vi "MakeDoor.vi"(7 "DoorID":T1, 8 "error in (no error)":errorcluster, 9 "Room 2":refnum<class "Room.lvclass">, 10 "Room 1":refnum<class "Room.lvclass">, 11 "MazeGame":refnum<class "MazeGame.lvclass">) -> (0 "error out":errorcluster, 2 "Door":refnum<class "Door.lvclass">, 3 "MazeGame":refnum<class "MazeGame.lvclass">)   [LabVIEW 2020, in "FactoryMethod.lvlib" / "ParameterizedFactoryMethod.lvlib" / "MazeGame.lvclass"]
uses:
  MazeGame.lvclass
  GoFcommonClasses/ConcreteMazeSite/Room/Room.lvclass
  GoFcommonClasses/ConcreteMazeSite/Door/Door.lvclass
  TypeDef/DoorID.ctl
  GoFcommonClasses/ConcreteMazeSite/DoorNeedingSpell/DoorNeedingSpell.lvclass
  E:/Francesco/GitHub/Design-Patterns-GoF_-_NI-LV/Creational/GoFcommonClasses/ConcreteMazeSite/Door/Door.lvclass
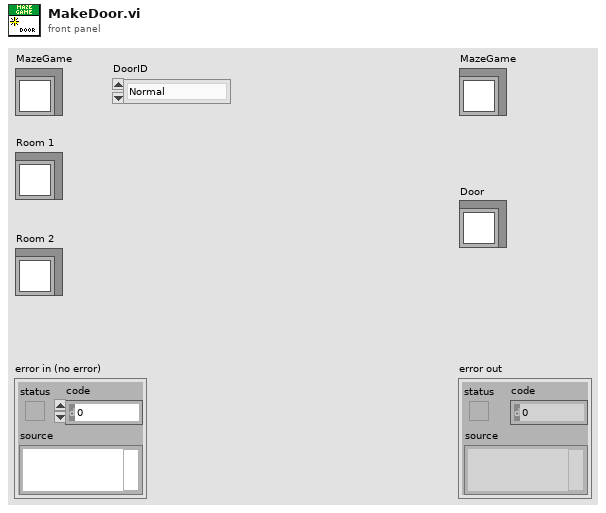
[diagram p1: front panel]
types:
  T1 = typedef "FactoryMethod.lvlib/ParameterizedFactoryMethod.lvlib/MazeGame.lvclass/DoorID.ctl" = enum8{"Normal", "Enchanted"}
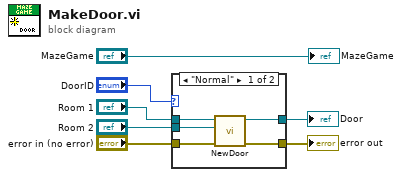
[diagram p0: block diagram]
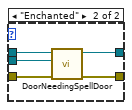
[diagram p2: hidden frame]
diagram:
  n1 = case shown="\"Normal\"" "DoorID" {
    tunnel: "Room 1" -> [w12 w14]
    tunnel: "Room 2" -> [w11 w13]
    tunnel: [w10 w15] -> w4
    tunnel: "error in (no error)" -> [w9 w17]
    tunnel: [w8 w16] -> w2
    frame "Normal" {
      n2 = call "NewDoor.vi"("error in (no error)"=w9, "Room 2"=w11, "Room 1"=w12) -> ("error out"=w8:errorcluster, "Door"=w10:refnum<class "Door.lvclass">)  [unwired: 7 in]
    }
    frame "Enchanted" {
      n3 = call "DoorNeedingSpellDoor.vi"("error in (no error)"=w17, "Room 2"=w13, "Room 1"=w14) -> ("error out"=w16:errorcluster, "DoorNeedingSpell"=w15:refnum<class "DoorNeedingSpell.lvclass">)  [unwired: 7 in]
    }
  }
  "error out" <- w2
  "Door" <- w4
  "MazeGame" <- "MazeGame"
